vi "Parse Current Projects Opened.vi"(8 "error in":errorcluster) -> (0 "error out":errorcluster, 3 "Current Projects Opened":string[](array[string]))   [LabVIEW 2020, in "Panther Dashboard.lvlib"]
uses:
  Panther Dashboard.lvlib
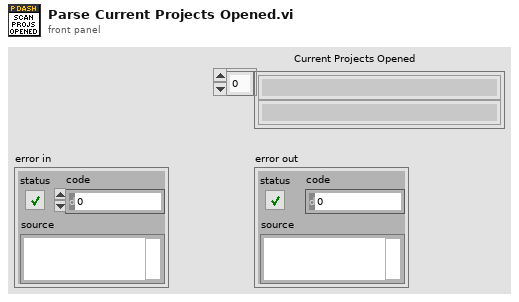
[diagram p1: front panel]
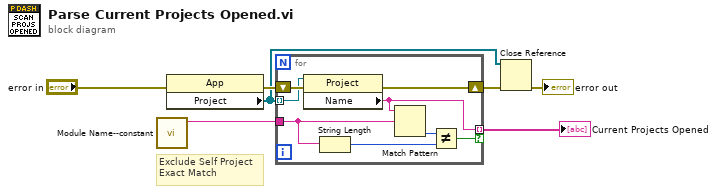
[diagram p0: block diagram]
diagram:
  # "Exclude Self Project\nExact Match"
  n1 = call "Module Name--constant.vi"() -> ("Module Name"=w1:string)  [unwired: 11 in]
  n2 = property class="App"(error in="error in") -> (error out=w5:errorcluster, "Project"=w2:refnum<vi>[])  [unwired: 1 in, 1 out]
  n3 = for {
    tunnel: w2 -> [w10] mode=indexing
    tunnel: [w13] -> w3 mode=indexing if=w11
    tunnel: w1 -> [w9]
    shift-right: [w15] -> w6
    shift-left: w5 -> [w14]
    n4 = property class="Project"(reference=w10, error in=w14) -> (error out=w15:errorcluster, "Name"=w13:string)  [unwired: 1 out]
    n5 = String Length(string=w9) -> (length=w8:i32)
    n6 = Match Pattern(string=w13, regular expression=w9) -> (offset past match=w12:i32)  [unwired: 1 in, 3 out]
    n7 = Not Equal?(x=w12, y=w8) -> (x != y?=w11:bool)
  }
  "Current Projects Opened" <- w3
  n8 = Close Reference(reference=w2, error in (no error)=w6) -> (error out=→"error out":errorcluster)
